vi "InTake Modifications.vi"(1 "InTake Global Data In":T1) -> (0 "InTake Global Data Out":T1)   [LabVIEW 2013]
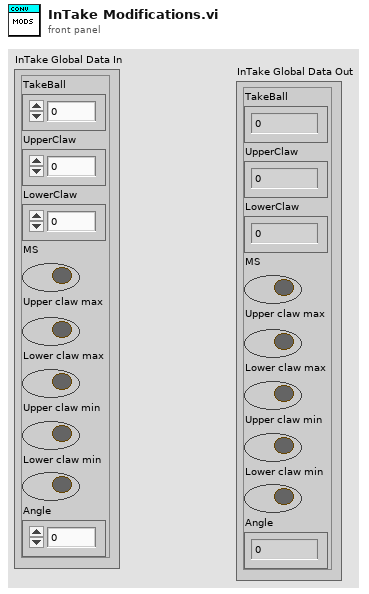
[diagram p1: front panel]
types:
  T1 = cluster{"TakeBall":dbl, "UpperClaw":dbl, "LowerClaw":dbl, "MS":bool, "Upper claw max":bool, "Lower claw max":bool, "Upper claw min":bool, "Lower claw min":bool, "Angle":dbl}
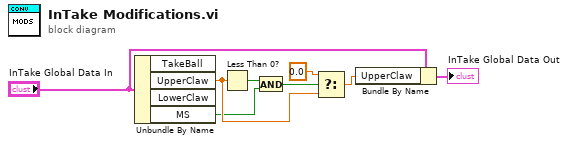
[diagram p0: block diagram]
diagram:
  n1 = Unbundle By Name("InTake Global Data In") -> ("UpperClaw"=w5:dbl, "MS"=w2:bool)  [unwired: 2 out]
  n2 = Less Than 0?(x=w5) -> (x < 0?=w1:bool)
  n3 = And(x=w1, y=w2) -> (x .and. y?=w6:bool)
  n4 = Select(t=0.0, s=w6, f=w5) -> (s? t:f=w3:dbl)
  n5 = Bundle By Name(cluster="InTake Global Data In", "UpperClaw"=w3) -> (→"InTake Global Data Out":T1)
